vi "Calibration.vi"() -> ()   [LabVIEW 2015]
uses:
  <vilib>/Analysis/baseanly.llb/Mean (DBL).vi
  <vilib>/Analysis/NI_AALBase.lvlib
panel:
  out "Pickup voltage amplitude, V":dbl format="%#_13g"
  out "Solenoid current amplitude, A":dbl format="%#_13g"
  out "Solenoid current (current sensor 0.1 Ohm)":cluster{"Array":dbl[], "Array 2":dbl[]}(graph)
  in  "Solenoild diameter, mm":dbl=6.0 format="%#_13g"
  out "Voltage to Gauss coefficient, V*s/(G*rad*m^2)":dbl format="%#_13g"
  in  "Solenoid wire diameter, mm":dbl=0.15 format="%#_13g"
  out "Pickup voltage":cluster{"Array":dbl[], "Array 2":dbl[]}(graph)
  in  "Number of periods":i32=100
  in  "Generator frequency, Hz":dbl=100.0 format="%#_13g"
  in  "DAQ sampling rate":dbl=100000.0 format="%#_13g"
  # "Connect the current sensor and the pickup coil to DAQ's channels 1 and 3 respectively"
  # "Yujie Zhao & Dmitriy Makhnovskiy\nJune 2019, Hangzhou, China"
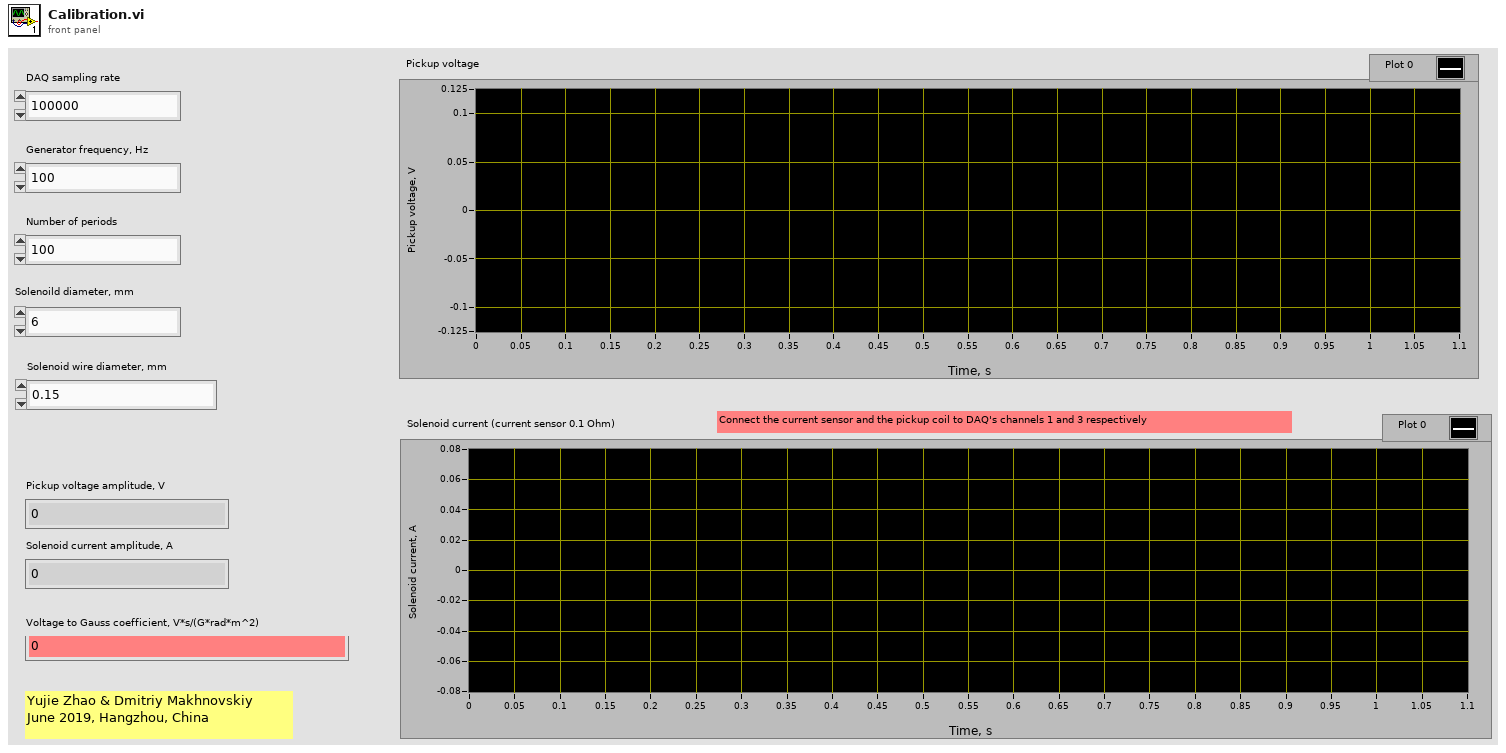
[diagram p1: front panel]
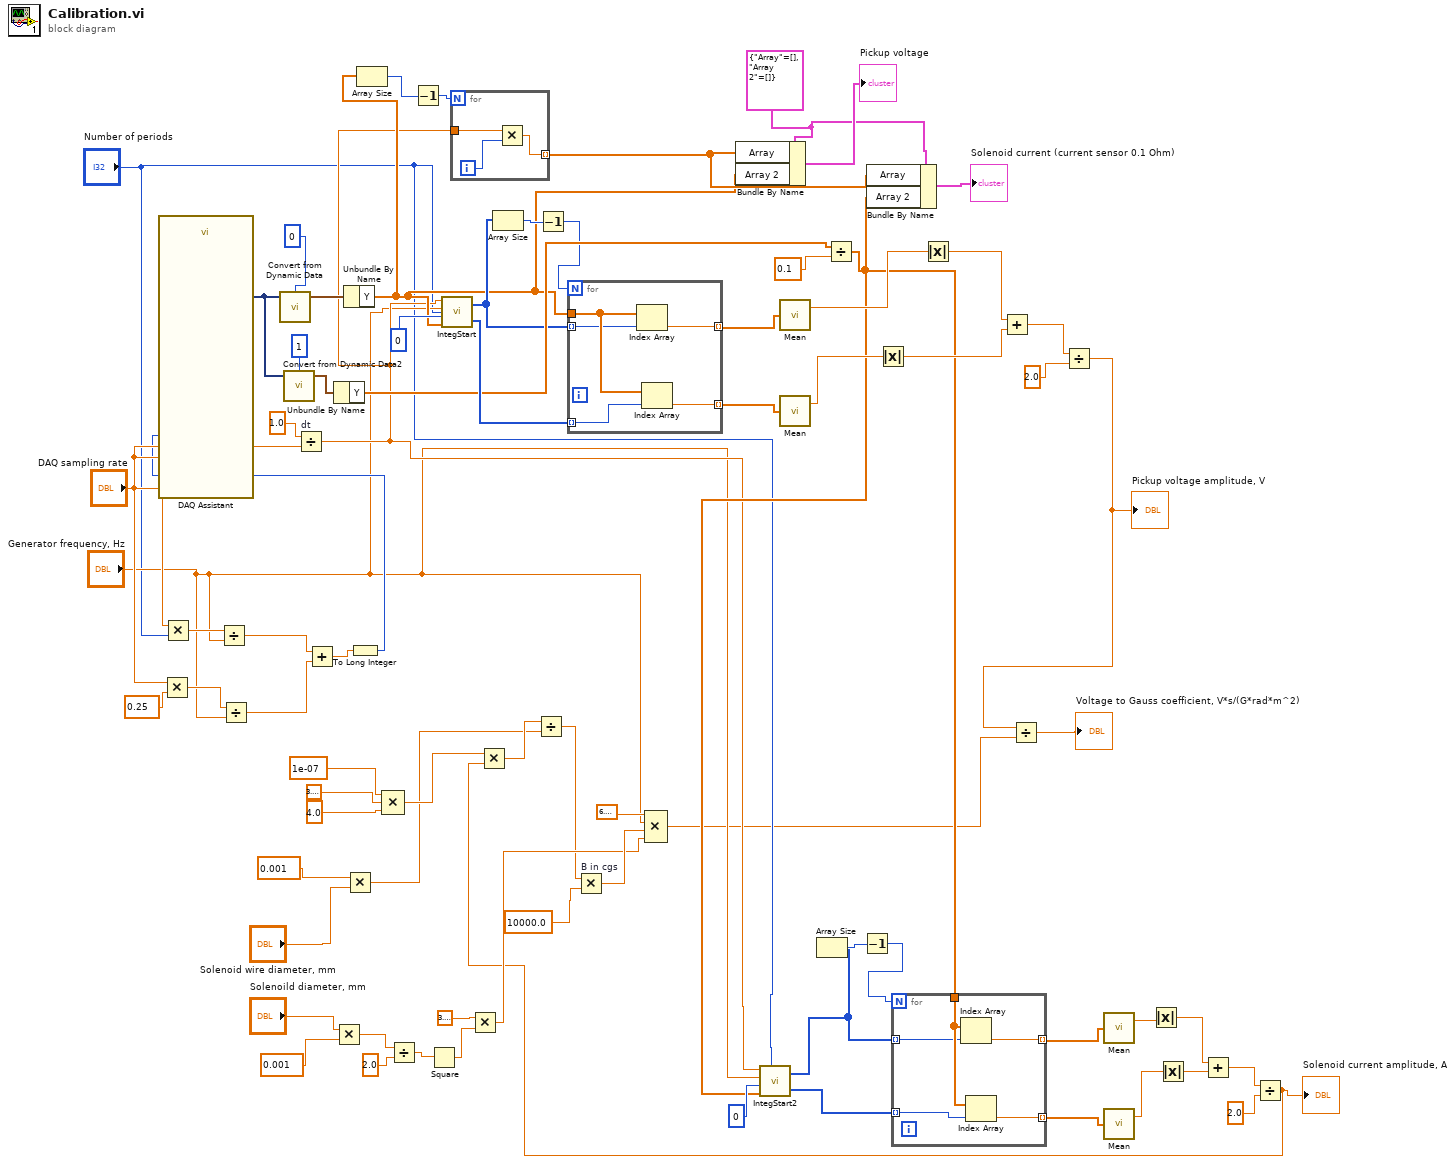
[diagram p0: block diagram]
diagram:
  w45 = cluster{"Array":dbl[], "Array 2":dbl[]} {"Array"=[], "Array 2"=[]} ("Cluster")
  n1 = Multiply(x="DAQ sampling rate", y=0.25) -> (x*y=w71:dbl)
  n2 = Multiply(x="DAQ sampling rate", y="Number of periods") -> (x*y=w75:dbl)
  n3 = Divide(x=w75, y="Generator frequency, Hz") -> (x/y=w74:dbl)
  n4 = Divide(x=w71, y="Generator frequency, Hz") -> (x/y=w70:dbl)
  n5 = Divide "dt"(x=1.0, y="DAQ sampling rate") -> (x/y=w8:dbl)
  n6 = Add(x=w74, y=w70) -> (x+y=w69:dbl)
  n7 = Multiply(x="Solenoild diameter, mm", y=0.001) -> (x*y=w52:dbl)
  n8 = Multiply(x=0.001, y="Solenoid wire diameter, mm") -> (x*y=w21:dbl)
  n9 = To Long Integer(number=w69) -> (32bit integer=w67:i32)
  n10 = call "DAQ Assistant"("rate"="DAQ sampling rate", "number of samples"=w67) -> ("data"=w42:dynamicdata)  [unwired: 15 in, 2 out]
  n11 = call "Convert from Dynamic Data"("Dynamic Data Type"=w42, "Channel"=0) -> ("Waveform"=w77:waveform(dbl))  [unwired: 2 in]
  n12 = call "Convert from Dynamic Data2"("Dynamic Data Type"=w42, "Channel"=1) -> ("Waveform"=w40:waveform(dbl))  [unwired: 2 in]
  n13 = Unbundle By Name(w40) -> ("Y"=w31:dbl[])
  n14 = Unbundle By Name(w77) -> ("Y"=w13:dbl[])
  n15 = Array Size(array=w13) -> (size(s)=w62:i32)
  n16 = Compound Arithmetic op=MULTIPLY(1e-07, 3.141592653589793, 4.0) -> (w38:dbl)
  n17 = Divide(x=w52, y=2.0) -> (x/y=w49:dbl)
  n18 = Decrement(x=w62) -> (x-1=w61:i32)
  n19 = Square(x=w49) -> (x^2=w48:dbl)
  n20 = call "IntegStart.vi"("Time step"=w8, "Generator frequency"="Generator frequency, Hz", "Number of ignored periods"=0, "Field"=w13, "BH averages"="Number of periods") -> ("Min Index"=w14:i32[], "Max Index"=w66:i32[])
  n21 = for {
    N: w61 -> [_]
    tunnel: w8 -> [w79]
    tunnel: [w78] -> w43 mode=indexing
    i -> [w80]
    n22 = Multiply(x=w79, y=w80) -> (x*y=w78:dbl)
  }
  n23 = Multiply(x=3.141592653589793, y=w48) -> (x*y=w47:dbl)
  n24 = Array Size(array=w14) -> (size(s)=w16:i32)
  n25 = Decrement(x=w16) -> (x-1=w12:i32)
  n26 = for {
    N: w12 -> [_]
    tunnel: w13 -> [w83]
    tunnel: w14 -> [w81] mode=indexing
    tunnel: [w82] -> w15 mode=indexing
    tunnel: w66 -> [w85] mode=indexing
    tunnel: [w84] -> w18 mode=indexing
    n27 = Index Array(array=w83, index=w81) -> (element=w82:dbl)
    n28 = Index Array(array=w83, index=w85) -> (element=w84:dbl)
  }
  n29 = Bundle By Name(cluster=w45, "Array"=w43, "Array 2"=w13) -> (→"Pickup voltage":cluster{"Array":dbl[], "Array 2":dbl[]})
  n30 = call-poly <vilib>:"Mean.vi"("X"=w15) -> ("mean"=w19:dbl)  [unwired: 1 out]
  n31 = call-poly <vilib>:"Mean.vi"("X"=w18) -> ("mean"=w17:dbl)  [unwired: 1 out]
  n32 = Divide(x=w31, y=0.1) -> (x/y=w9:dbl[])
  n33 = call "IntegStart2.vi"("Time step"=w8, "Generator frequency"="Generator frequency, Hz", "Number of ignored periods"=0, "Field"=w9, "BH averages"="Number of periods") -> ("Min Index"=w5:i32[], "Max Index"=w4:i32[])
  n34 = Array Size(array=w5) -> (size(s)=w33:i32)
  n35 = Decrement(x=w33) -> (x-1=w11:i32)
  n36 = Bundle By Name(cluster=w45, "Array"=w43, "Array 2"=w9) -> (→"Solenoid current (current sensor 0.1 Ohm)":cluster{"Array":dbl[], "Array 2":dbl[]})
  n37 = Absolute Value(x=w17) -> (abs(x)=w20:dbl)
  n38 = for {
    N: w11 -> [_]
    tunnel: w5 -> [w86] mode=indexing
    tunnel: [w90] -> w35 mode=indexing
    tunnel: [w89] -> w34 mode=indexing
    tunnel: w9 -> [w88]
    tunnel: w4 -> [w87] mode=indexing
    n39 = Index Array(array=w88, index=w86) -> (element=w90:dbl)
    n40 = Index Array(array=w88, index=w87) -> (element=w89:dbl)
  }
  n41 = Absolute Value(x=w19) -> (abs(x)=w65:dbl)
  n42 = Add(x=w65, y=w20) -> (x+y=w63:dbl)
  n43 = Divide(x=w63, y=2.0) -> (x/y=w1:dbl)
  "Pickup voltage amplitude, V" <- w1
  n44 = call-poly <vilib>:"Mean.vi"("X"=w35) -> ("mean"=w30:dbl)  [unwired: 1 out]
  n45 = call-poly <vilib>:"Mean.vi"("X"=w34) -> ("mean"=w26:dbl)  [unwired: 1 out]
  n46 = Absolute Value(x=w30) -> (abs(x)=w29:dbl)
  n47 = Absolute Value(x=w26) -> (abs(x)=w25:dbl)
  n48 = Add(x=w29, y=w25) -> (x+y=w28:dbl)
  n49 = Divide(x=w28, y=2.0) -> (x/y=w24:dbl)
  "Solenoid current amplitude, A" <- w24
  n50 = Multiply(x=w38, y=w24) -> (x*y=w37:dbl)
  n51 = Divide(x=w37, y=w21) -> (x/y=w36:dbl)
  n52 = Multiply "B in cgs"(x=w36, y=10000.0) -> (x*y=w55:dbl)
  n53 = Compound Arithmetic op=MULTIPLY(6.283185307179586, "Generator frequency, Hz", w55, w47) -> (w2:dbl)
  n54 = Divide(x=w1, y=w2) -> (x/y=→"Voltage to Gauss coefficient, V*s/(G*rad*m^2)":dbl)
